vi "Array-Index of Last Element.vi"(1 "Array":dbl[](array[numeric])) -> (0 "Last Index":i32)   [LabVIEW 2020]
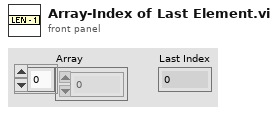
[diagram p1: front panel]
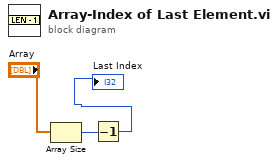
[diagram p0: block diagram]
diagram:
  n1 = Array Size(array="Array") -> (size(s)=w2:i32)
  n2 = Decrement(x=w2) -> (x-1=→"Last Index":i32)
